vi "Read Key Tap.vi"   [LabVIEW 2014, in "LMH-Leap.lvlib"]
doc: "Read all data from key tap gestures. Use the polymorphic instance to select between one or N key tap gestures."
uses:
  LMH-Leap.lvlib
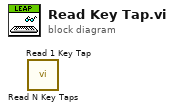
[diagram p0: block diagram]
diagram:
  n1 = call "Read N Key Taps.vi"() -> ()  [unwired: 8 in, 4 out]
  n2 = call "Read 1 Key Tap.vi"() -> ()  [unwired: 8 in, 4 out]
